vi "PointerSize.vi"() -> (0 "Pointer Size [Byte]":i32)   [LabVIEW 2024, in "SDL3.lvlib" / "LV-Utilities.lvlib"]
uses:
  LV-Utilities.lvlib
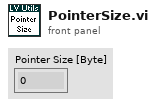
[diagram p1: front panel]
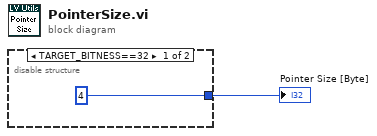
[diagram p0: block diagram]
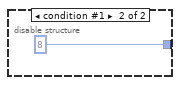
[diagram p2: hidden frame]
diagram:
  n1 = disable-structure shown="TARGET_BITNESS==32" {
    disable-tunnel: [4 ("Size") 8 ("Size")] -> w1
    frame condition #0 (active) {
    }
    frame condition #1 {
    }
  }
  "Pointer Size [Byte]" <- w1
